vi "Get Item Display Name.vi"(8 "error in (no error)":errorcluster, 9 "Tag":string, 11 "TreeControl in":refnum<vi>) -> (0 "error out":errorcluster, 1 "index":i32, 2 "display name":string, 3 "TreeControl out":refnum<vi>)   [LabVIEW 2019, in "DSF Configuration Utility.lvlib"]
uses:
  DSF Configuration Utility.lvlib
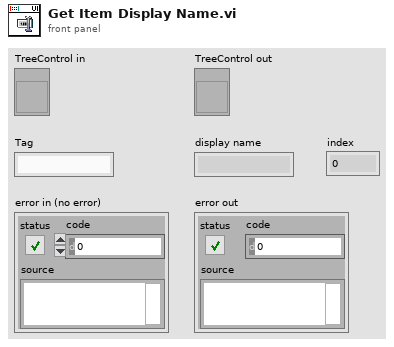
[diagram p1: front panel]
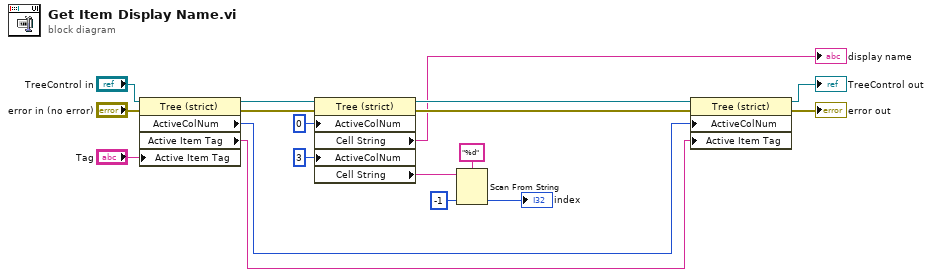
[diagram p0: block diagram]
diagram:
  n1 = property class="Tree (strict)"(reference="TreeControl in", error in="error in (no error)", "Active Item Tag"="Tag") -> (reference out=w12:refnum<vi>, error out=w15:errorcluster, "ActiveColNum"=w14:i32, "Active Item Tag"=w9:string)
  n2 = property class="Tree (strict)"(reference=w12, error in=w15, "ActiveColNum"=0 ("Active Cell:Active Column Number"), "ActiveColNum"=3 ("Active Cell:Active Column Number")) -> (reference out=w13:refnum<vi>, error out=w16:errorcluster, "Cell String"=→"display name":string, "Cell String"=w1:string)
  n3 = Scan From String(format string="%d", input string=w1, default 1=-1 ("default value 1")) -> (output 1=→"index":i32)  [unwired: 2 in, 3 out]
  n4 = property class="Tree (strict)"(reference=w13, error in=w16, "ActiveColNum"=w14, "Active Item Tag"=w9) -> (reference out=→"TreeControl out":refnum<vi>, error out=→"error out":errorcluster)
